vi "YKPZ400 Main.vi"(8 "error in (no error)":errorcluster, 9 "Metadata all":T1={"Data Fields"={"operatorName"="LED Life Testing", "project"="LED Life Testing", "measurementType"="", "sphere"="2m (jacketed)", "spectrometer"="", "powerSource"="California Instruments 2253ix", "analyzer"="California Instruments 2253ix", "fixtureType"="NA", "lampType"="A 19", "sourceType"="LED", "testOrientation"="Base Up", "model"="1", "sample"="1", "hours"="1000", "Amp Gain Range"=""}, "Metadata Disable"={"spectrometer"=enum."Disabled and Grayed Out", "sphere"=enum."Disabled and Grayed Out", "analyzer"=enum."Disabled and Grayed Out", "ampGainRange"=enum."Disabled and Grayed Out"}, "Output Path"=path ""}, 10 "Master":refnum<queue>, 11 "Stand alone?":bool) -> (0 "error out":errorcluster)   [LabVIEW 2013, in "Yokogawa.lvlib"]
doc: "This Continuous Measurement sample project is based on the Queued Message Handler template.\n\nThe Event Handling Loop generates messages based on user interface actions.\n\nThe Message Handling Loop processes messages generated by the Event Handling Loop, or by other messages. There are also Acquisition and Logging message handling loop subVIs, and a chart updating loop."
uses:
  Yokogawa.lvlib
  controls/electrical2.ctl
  support/Message Queue/Message Cluster.ctl
  controls/Metadata all typedef.ctl
  controls/Metadata typedef.ctl
  controls/Metadata disable typedef.ctl
  Settings/Settings.ctl
  Acquisition/Hardware Configuration.ctl
  Logging/Logging Configuration.ctl
  controls/YKPZ400 UI Data.ctl
  controls/YKPZ400 UI State.ctl
  support/Message Queue/Enqueue Message (Single).vi
  support/Message Queue/Enqueue Message (Array).vi
  <vilib>/Utility/error.llb/Error Cluster From Error Code.vi
  <vilib>/ErrorRing/Error Ring.xnode
  Acquisition/YKPZ400 Acquisition.lvlib
  Logging/YKPZ400 Logging.lvlib
  Settings/YKPZ400 Settings.lvlib
  support/User Event - Stop/YKPZ400 User Event - Stop.lvlib
  support/Message Queue/YKPZ400 Message Queue.lvlib
panel:
  out "Electrical Data":T4
  in  "Save Data":bool
  in  "Settings":bool
  in  "Start":bool
  in  "Stop":bool
  in  "Exit":bool
  out "Status":string
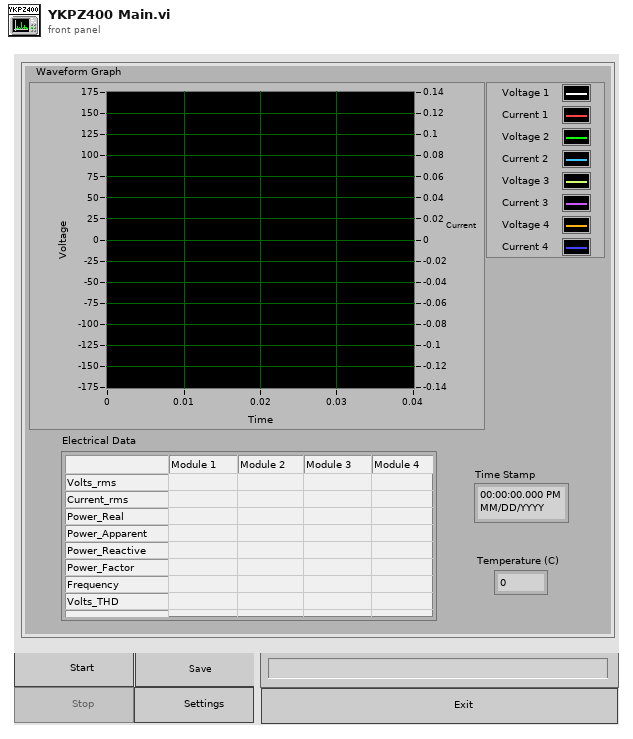
[diagram p1: front panel]
types:
  T1 = typedef "Yokogawa.lvlib/YKPZ400 Logging.lvlib/Metadata all typedef.ctl" = cluster{"Data Fields":T2, "Metadata Disable":T3, "Output Path":path}
  T2 = typedef "Yokogawa.lvlib/YKPZ400 Logging.lvlib/Metadata typedef.ctl" = cluster{"operatorName":string, "project":string, "measurementType":string, "sphere":string, "spectrometer":string, "powerSource":string, "analyzer":string, "fixtureType":string, "lampType":string, "sourceType":string, "testOrientation":string, "model":string, "sample":string, "hours":string, "Amp Gain Range":string}
  T3 = typedef "Yokogawa.lvlib/YKPZ400 Logging.lvlib/Metadata disable typedef.ctl" = cluster{"spectrometer":enum8{"Enabled", "Disabled", "Disabled and Grayed Out"}, "sphere":enum8{"Enabled", "Disabled", "Disabled and Grayed Out"}, "analyzer":enum8{"Enabled", "Disabled", "Disabled and Grayed Out"}, "ampGainRange":enum8{"Enabled", "Disabled", "Disabled and Grayed Out"}}
  T4 = typedef "Yokogawa.lvlib/YKPZ400 Acquisition.lvlib/electrical2.ctl" = cluster{"Time Stamp":timestamp, "Temperature (C)":dbl, "Electrical Data":string[][], "Waveform Graph":waveform(dbl)[]}
  T5 = typedef "Yokogawa.lvlib/YKPZ400 UI State.ctl" = enum16{"Idle", "Acquiring and Logging", "Waiting for Exit", "Waiting for Exit (Acq Stopped)", "Waiting for Exit (Log Stopped)", "Waiting for Stop", "Waiting for Stop (Acq Stopped)", "Waiting for Stop (Log Stopped)"}
  T6 = typedef "Yokogawa.lvlib/YKPZ400 UI Data.ctl" = cluster{"Start Ref":refnum<vi>, "Stop Ref":refnum<vi>, "Settings Ref":refnum<vi>, "Exit Ref":refnum<vi>, "Status Ref":refnum<vi>, "Clust Refnum":refnum<vi>, "Save Refnum":refnum<vi>}
  T7 = typedef "Yokogawa.lvlib/YKPZ400 Settings.lvlib/Settings.ctl" = cluster{"Hardware Configuration":T8, "Logging Configuration":T9}
  T8 = typedef "Yokogawa.lvlib/YKPZ400 Acquisition.lvlib/Hardware Configuration.ctl" = cluster{"VISA resource name":refnum<visa-resource-name>, "Mode (0: Normal) ":u16, "Voltage":cluster{"Element (0: All)":u16, "V Range (200)":u16}, "Current":cluster{"A Range (2)":u16, "A Terminal (0: 5A)":u16, "Element (0: ALL)":u16}, "Observation Time":u16, "Modules on/off":cluster{"Module 1":bool, "Module 2":bool, "Module 3":bool, "Module 4":bool}}
  T9 = typedef "Yokogawa.lvlib/YKPZ400 Logging.lvlib/Logging Configuration.ctl" = cluster{"Log File Base Path":path, "TDMS File Reference":refnum<k34>, "Module to save":i32}
  T10 = typedef "Yokogawa.lvlib/YKPZ400 Message Queue.lvlib/All Message Queues.ctl" = cluster{"Master":refnum<queue>, "UI":refnum<queue>, "Acquisition":refnum<queue>, "Logging":refnum<queue>}
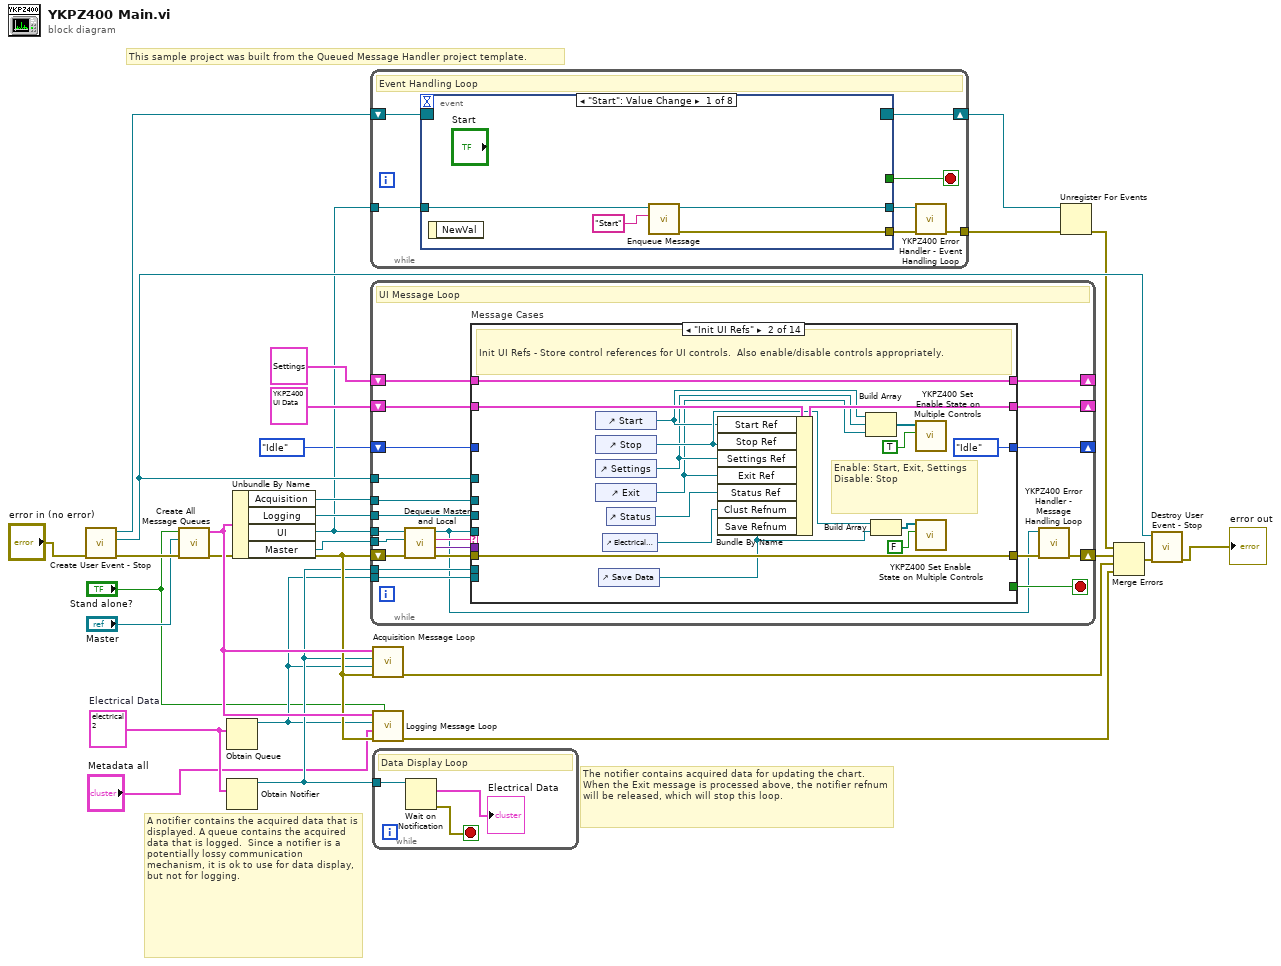
[diagram p0: block diagram]
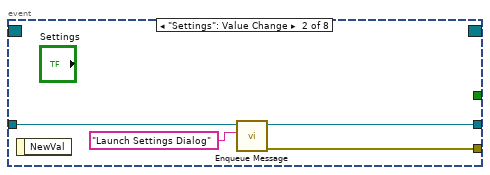
[diagram p2: hidden frame]
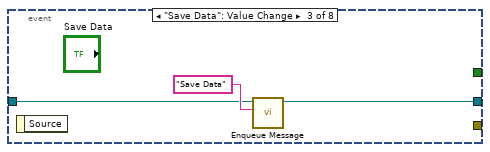
[diagram p3: hidden frame]
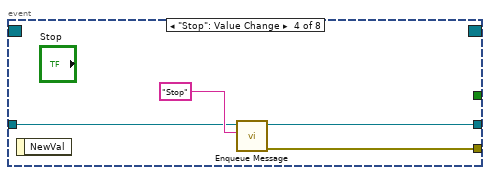
[diagram p4: hidden frame]
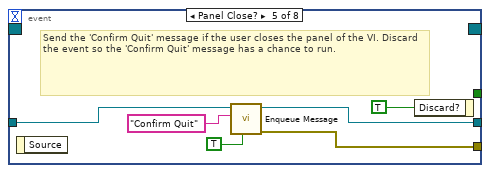
[diagram p5: hidden frame]
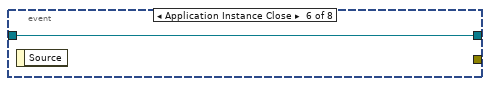
[diagram p6: hidden frame]
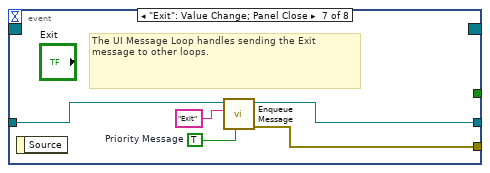
[diagram p7: hidden frame]
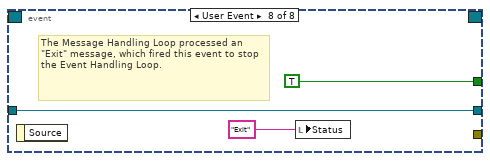
[diagram p8: hidden frame]
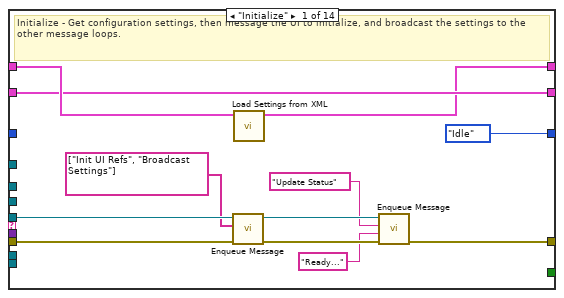
[diagram p9: hidden frame]
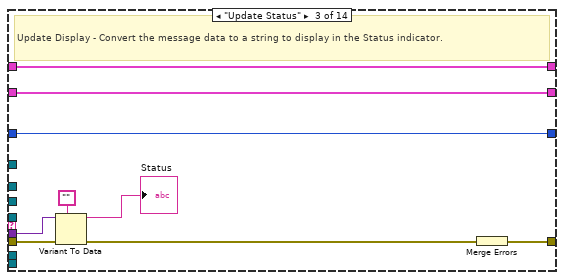
[diagram p10: hidden frame]
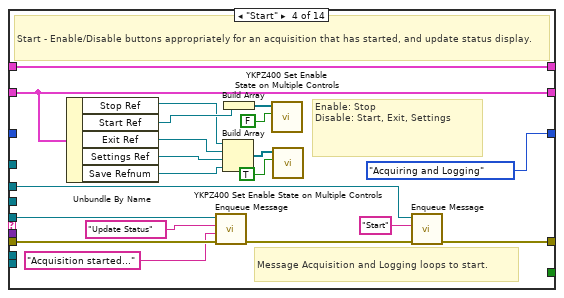
[diagram p11: hidden frame]
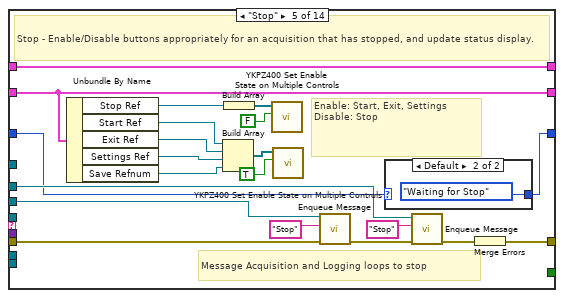
[diagram p12: hidden frame]
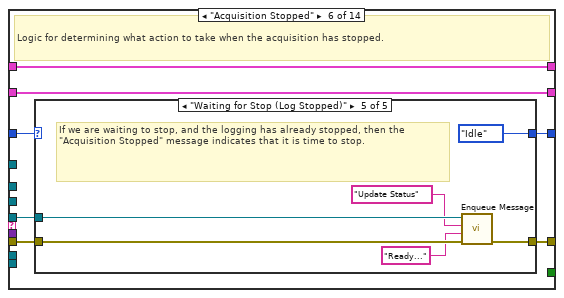
[diagram p14: hidden frame]
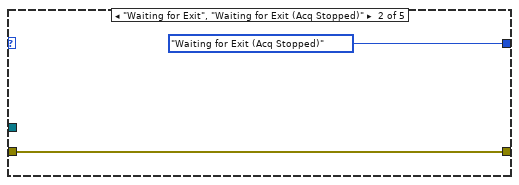
[diagram p16: hidden frame]
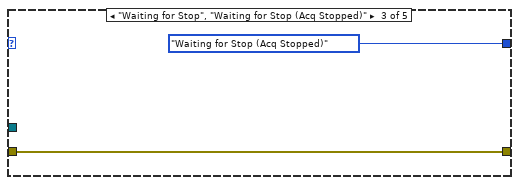
[diagram p17: hidden frame]
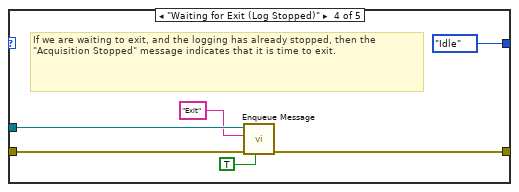
[diagram p18: hidden frame]
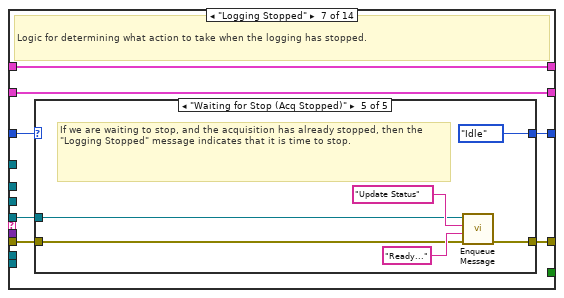
[diagram p19: hidden frame]
diagram:
  w9 = T4 {"Time Stamp"=timestamp(0 s since 1904-01-01), "Temperature (C)"=0.0, "Electrical Data"=[], "Waveform Graph"=[]}  # Electrical Data
  # "This sample project was built from the Queued Message Handler project template."
  # "A notifier contains the acquired data that is displayed. A queue contains the acquired data that is logged.  Since a notifier is a potentially lossy communication mechanism, it is ok to use for data display, but not for logging."
  # "The notifier contains acquired data for updating the chart. When the Exit message is processed above, the notifier refnum will be released, which will stop this loop."
  n1 = call "Create User Event - Stop.vi"("error in (no error)"="error in (no error)") -> ("error out"=w22:errorcluster, "User Event - Stop"=w24:refnum<user-event>, "Stop Event Registration Refnum"=w25:refnum<event-registration>)  [unwired: 8 in]
  n2 = call "Create All Message Queues.vi"("error in (no error)"=w22, "Master"="Master", "Stand alone?"="Stand alone?") -> ("error out"=w19:errorcluster, "Message Queues out"=w21:T10)  [unwired: 7 in]
  n3 = Obtain Queue(element data type=w9) -> (queue out=w7:refnum<queue>)  [unwired: 4 in, 2 out]
  n4 = Obtain Notifier(notification data type=w9) -> (notifier out=w8:refnum<notifier>)  [unwired: 3 in, 2 out]
  n5 = Unbundle By Name(w21) -> ("Acquisition"=w14:refnum<queue>, "Logging"=w13:refnum<queue>, "UI"=w12:refnum<queue>, "Master"=w1:refnum<queue>)
  n6 = while {
    tunnel: w12 -> [w33]
    tunnel: [w30] -> w26
    shift-right: [w32] -> w16
    shift-left: w25 -> [w34]
    stop <- w31 stop-if-true
    # "Event Handling Loop"
    n7 = event shown="[0] \"Start\": Value Change" {
      selector: w34 -> [_ _ _ _ _ _ _ _]
      dyn-events: [_ _ _ _ _ _ _ _] -> w32
      timeout: _ -> [_ _ _ _ _ _ _ _]
      tunnel: [_ _ _ _ _ _ _ TRUE ("Discard?")] -> w31
      tunnel: w33 -> [w38 w40 w44 w48 w53 w56 w58 w62]
      tunnel: [w36 w42 _ w47 w51 _ w61 _] -> w29
      tunnel: [w35 w39 w43 w46 w52 w56 w57 w62] -> w28
      event "Start": Value Change {
        n8 = event-data() -> ()  [unwired: 1 in, 1 out]
        n9 = call-poly "Enqueue Message.vi"("Message"="Start", "Message Queue"=w38) -> ("error out"=w36:errorcluster, "dup Message Queue"=w35:refnum<queue>)  [unwired: 8 in]
      }
      event "Settings": Value Change {
        n10 = event-data() -> ()  [unwired: 1 in, 1 out]
        n11 = call-poly "Enqueue Message.vi"("Message"="Launch Settings Dialog", "Message Queue"=w40) -> ("error out"=w42:errorcluster, "dup Message Queue"=w39:refnum<queue>)  [unwired: 8 in]
      }
      event "Save Data": Value Change {
        n12 = event-data() -> ()  [unwired: 1 in, 1 out]
        n13 = call-poly "Enqueue Message.vi"("Message"="Save Data", "Message Queue"=w44) -> ("dup Message Queue"=w43:refnum<queue>)  [unwired: 8 in, 1 out]
      }
      event "Stop": Value Change {
        n14 = event-data() -> ()  [unwired: 1 in, 1 out]
        n15 = call-poly "Enqueue Message.vi"("Message"="Stop", "Message Queue"=w48) -> ("error out"=w47:errorcluster, "dup Message Queue"=w46:refnum<queue>)  [unwired: 8 in]
      }
      event Panel Close? {
        # "Send the 'Confirm Quit' message if the user closes the panel of the VI. Discard the event so the 'Confirm Quit' message has a chance to run."
        n16 = event-data() -> ()  [unwired: 1 in, 1 out]
        n17 = call-poly "Enqueue Message.vi"("Priority Message? (F)"=TRUE, "Message"="Confirm Quit", "Message Queue"=w53) -> ("error out"=w51:errorcluster, "dup Message Queue"=w52:refnum<queue>)  [unwired: 7 in]
        n18 = event-data("Discard?"=TRUE) -> ()  [unwired: 1 in, 1 out]
      }
      event Application Instance Close {
        n19 = event-data() -> ()  [unwired: 1 in, 1 out]
      }
      event "Exit": Value Change; Panel Close {
        w59 = TRUE  # Priority Message
        # "The UI Message Loop handles sending the Exit message to other loops."
        n20 = event-data() -> ()  [unwired: 1 in, 1 out]
        n21 = call-poly "Enqueue Message.vi"("Priority Message? (F)"=w59, "Message"="Exit", "Message Queue"=w58) -> ("error out"=w61:errorcluster, "dup Message Queue"=w57:refnum<queue>)  [unwired: 7 in]
      }
      event User Event {
        # "The Message Handling Loop processed an \"Exit\" message, which fired this event to stop the Event Handling Loop."
        n22 = event-data() -> ()  [unwired: 1 in, 1 out]
        n23 = local write "Status"("Exit" ("Exit String")) -> ()
      }
    }
    n24 = call "YKPZ400 Error Handler - Event Handling Loop.vi"("error in (no error)"=w29, "Message Queue"=w28) -> ("dup error in"=w30:errorcluster)  [unwired: 8 in, 1 out]
  }
  n25 = while {
    tunnel: w12 -> [w71]
    tunnel: w24 -> [w84]
    shift-right: [w75] -> w27
    shift-left: w19 -> [w69]
    shift-right: [w83] -> _
    shift-left: T7 {"Hardware Configuration"={"VISA resource name"="", "Mode (0: Normal) "=0, "Voltage"={"Element (0: All)"=0, "V Range (200)"=0}, "Current"={"A Range (2)"=0, "A Terminal (0: 5A)"=0, "Element (0: ALL)"=0}, "Observation Time"=0, "Modules on/off"={"Module 1"=FALSE, "Module 2"=FALSE, "Module 3"=FALSE, "Module 4"=FALSE}}, "Logging Configuration"={"Log File Base Path"=path "", "TDMS File Reference"=refnum, "Module to save"=0}} ("Settings") -> [w82]
    shift-right: [w80] -> _
    shift-left: T6 {"Start Ref"=refnum, "Stop Ref"=refnum, "Settings Ref"=refnum, "Exit Ref"=refnum, "Status Ref"=refnum, "Clust Refnum"=refnum, "Save Refnum"=refnum} ("Measurement UI Controls") -> [w81]
    tunnel: w14 -> [w79]
    tunnel: w13 -> [w78]
    tunnel: w8 -> [w77]
    tunnel: w7 -> [w76]
    shift-right: [w72] -> _
    shift-left: YKPZ400_UI_State."Idle" ("UI State") -> [w73]
    tunnel: w1 -> [w70]
    stop <- w85 stop-if-true
    # "UI Message Loop"
    n26 = call "Dequeue Master and Local.vi"("error in (no error)"=w69, "Master"=w70, "UI In"=w71) -> ("error out"=w67:errorcluster, "Message Data"=w68:variant, "Message"=w66:string, "UI Out"=w65:refnum<queue>)  [unwired: 5 in]
    n27 = case "Message Cases" shown="\"Init UI Refs\"" w66 {
      selector: w66 -> [_ _ _ _ _ _ _ _ _ _ _ _ _ w313]
      tunnel: w65 -> [w90 _ _ w142 _ w168 w193 _ w233 w247 w258 w289 w303 _]
      tunnel: w67 -> [w89 w113 w121 w141 w162 w169 w194 w221 w235 w250 w257 w297 w301 _]
      tunnel: [w94 w113 w122 w130 w163 w166 w191 w227 w230 w246 w256 w298 w311 w312] -> w74
      tunnel: [_ _ _ _ _ _ _ _ _ _ _ TRUE _ _] -> w85
      tunnel: w68 -> [_ _ w120 _ _ _ _ _ _ w248 _ _ _ _]
      tunnel: w84 -> [_ _ _ _ _ _ _ _ _ _ _ w296 _ _]
      tunnel: [w86 w112 w116 w140 w161 w172 w197 w225 w232 w254 w261 w294 w310 w316] -> w83
      tunnel: w82 -> [w97 w112 w116 w140 w161 w172 w197 w225 w236 w254 w261 w294 w310 w316]
      tunnel: w81 -> [w91 w111 w115 w137 w160 w171 w196 w219 w229 w253 w260 w292 w309 w315]
      tunnel: [w91 w109 w115 w137 w160 w171 w196 w219 w229 w253 w260 w292 w309 w315] -> w80
      tunnel: w79 -> [_ _ _ w129 w147 _ _ w218 _ _ _ w291 _ _]
      tunnel: w78 -> [_ _ _ _ w150 _ _ w217 _ _ _ w290 w306 _]
      tunnel: w77 -> [_ _ _ _ _ _ _ _ _ _ _ w288 _ _]
      tunnel: w76 -> [_ _ _ _ _ _ _ _ _ _ _ w284 _ _]
      tunnel: w73 -> [_ _ w114 _ w144 w170 w195 w216 w228 w242 w259 _ w308 w314]
      tunnel: [YKPZ400_UI_State."Idle" ("UI State") YKPZ400_UI_State."Idle" ("UI State") w114 YKPZ400_UI_State."Acquiring and Logging" ("UI State") w145 w167 w192 w216 w228 w242 w255 YKPZ400_UI_State."Idle" ("UI State") w308 w314] -> w72
      frame "Initialize" {
        # "Initialize - Get configuration settings, then message the UI to initialize, and broadcast the settings to the other message loops."
        n28 = call-poly "Enqueue Message.vi"("error in (no error)"=w89, "Message Array"=string[] ["Init UI Refs", "Broadcast Settings"], "Message Queue"=w90) -> ("error out"=w96:errorcluster, "dup Message Queue"=w95:refnum<queue>)  [unwired: 7 in]
        n29 = call "Load Settings from XML.vi"("Settings in"=w97) -> ("Settings out"=w86:T7)  [unwired: 9 in, 1 out]
        n30 = call-poly "Enqueue Message.vi"("error in (no error)"=w96, "Message Data"="Ready..." ("Ready..."), "Message"="Update Status", "Message Queue"=w95) -> ("error out"=w94:errorcluster)  [unwired: 6 in, 1 out]
      }
      frame "Init UI Refs" {
        # "Enable: Start, Exit, Settings\nDisable: Stop"
        # "Init UI Refs - Store control references for UI controls.  Also enable/disable controls appropriately."
        n31 = control-ref of="Start"() -> (w103:refnum<vi>)
        n32 = control-ref of="Stop"() -> (w104:refnum<vi>)
        n33 = control-ref of="Settings"() -> (w102:refnum<vi>)
        n34 = control-ref of="Exit"() -> (w101:refnum<vi>)
        n35 = control-ref of="Save Data"() -> (w98:refnum<vi>)
        n36 = control-ref of="Electrical Data 2"() -> (w99:refnum<vi>)
        n37 = control-ref of="Status"() -> (w110:refnum<vi>)
        n38 = Bundle By Name(cluster=w111, "Start Ref"=w103, "Stop Ref"=w104, "Settings Ref"=w102, "Exit Ref"=w101, "Status Ref"=w110, "Clust Refnum"=w99, "Save Refnum"=w98) -> (w109:T6)
        n39 = Build Array(w103, w102, w101) -> (w107:refnum<vi>[])
        n40 = Build Array(w104, w98) -> (w106:refnum<vi>[])
        n41 = call "YKPZ400 Set Enable State on Multiple Controls.vi"("Enable?"=TRUE, "Controls"=w107) -> ()  [unwired: 10 in]
        n42 = call "YKPZ400 Set Enable State on Multiple Controls.vi"("Enable?"=FALSE, "Controls"=w106) -> ()  [unwired: 10 in]
      }
      frame "Update Status" {
        # "Update Display - Convert the message data to a string to display in the Status indicator."
        n43 = Variant To Data(error in=w121, type="", Variant=w120) -> (data=→"Status":string, error out=w118:errorcluster)
        n44 = Merge Errors(w118) -> (w122:errorcluster)
      }
      frame "Start" {
        # "Message Acquisition and Logging loops to start."
        # "Enable: Stop\nDisable: Start, Exit, Settings"
        # "Start - Enable/Disable buttons appropriately for an acquisition that has started, and update status display."
        n45 = Unbundle By Name(w137) -> ("Stop Ref"=w123:refnum<vi>, "Start Ref"=w124:refnum<vi>, "Exit Ref"=w132:refnum<vi>, "Settings Ref"=w131:refnum<vi>, "Save Refnum"=w125:refnum<vi>)
        n46 = call-poly "Enqueue Message.vi"("error in (no error)"=w141, "Message Data"="Acquisition started..." ("Acquiring and Logging..."), "Message"="Update Status", "Message Queue"=w142) -> ("error out"=w126:errorcluster)  [unwired: 6 in, 1 out]
        n47 = Build Array(w123, w132, w131, w125) -> (w135:refnum<vi>[])
        n48 = Build Array(w124) -> (w134:refnum<vi>[])
        n49 = call "YKPZ400 Set Enable State on Multiple Controls.vi"("Enable?"=FALSE, "Controls"=w134) -> ()  [unwired: 10 in]
        n50 = call "YKPZ400 Set Enable State on Multiple Controls.vi"("Enable?"=TRUE, "Controls"=w135) -> ()  [unwired: 10 in]
        n51 = call-poly "Enqueue Message.vi"("error in (no error)"=w126, "Message"="Start", "Message Queue"=w129) -> ("error out"=w130:errorcluster)  [unwired: 7 in, 1 out]
      }
      frame "Stop" {
        # "Message Acquisition and Logging loops to stop"
        # "Enable: Start, Exit, Settings\nDisable: Stop"
        # "Stop - Enable/Disable buttons appropriately for an acquisition that has stopped, and update status display."
        n52 = Unbundle By Name(w160) -> ("Stop Ref"=w155:refnum<vi>, "Start Ref"=w154:refnum<vi>, "Exit Ref"=w153:refnum<vi>, "Settings Ref"=w152:refnum<vi>, "Save Refnum"=w143:refnum<vi>)
        n53 = Build Array(w154, w153, w152, w143) -> (w158:refnum<vi>[])
        n54 = Build Array(w155) -> (w157:refnum<vi>[])
        n55 = call "YKPZ400 Set Enable State on Multiple Controls.vi"("Enable?"=FALSE, "Controls"=w157) -> ()  [unwired: 10 in]
        n56 = call "YKPZ400 Set Enable State on Multiple Controls.vi"("Enable?"=TRUE, "Controls"=w158) -> ()  [unwired: 10 in]
        n57 = call-poly "Enqueue Message.vi"("error in (no error)"=w162, "Message"="Stop", "Message Queue"=w150) -> ("error out"=w149:errorcluster)  [unwired: 7 in, 1 out]
        n58 = case shown="Default" w144 {
          selector: w144 -> [w164 _]
          tunnel: [w164 YKPZ400_UI_State."Waiting for Stop" ("UI State")] -> w145
          frame "Waiting for Exit" {
          }
          frame Default {
          }
        }
        n59 = call-poly "Enqueue Message.vi"("error in (no error)"=w149, "Message"="Stop", "Message Queue"=w147) -> ("error out"=w148:errorcluster)  [unwired: 7 in, 1 out]
        n60 = Merge Errors(w148) -> (w163:errorcluster)
      }
      frame "Acquisition Stopped" {
        # "Logic for determining what action to take when the acquisition has stopped."
        n61 = case shown="\"Waiting for Stop (Log Stopped)\"" w170 {
          selector: w170 -> [w174 _ _ _ _]
          tunnel: w169 -> [w173 w176 w178 w184 w190]
          tunnel: w168 -> [_ _ _ w182 w187]
          tunnel: [w174 YKPZ400_UI_State."Waiting for Exit (Acq Stopped)" ("UI State") YKPZ400_UI_State."Waiting for Stop (Acq Stopped)" ("UI State") YKPZ400_UI_State."Idle" ("UI State") YKPZ400_UI_State."Idle" ("UI State")] -> w167
          tunnel: [w173 w176 w178 w183 w188] -> w166
          frame Default {
          }
          frame "Waiting for Exit", "Waiting for Exit (Acq Stopped)" {
          }
          frame "Waiting for Stop", "Waiting for Stop (Acq Stopped)" {
          }
          frame "Waiting for Exit (Log Stopped)" {
            # "If we are waiting to exit, and the logging has already stopped, then the \"Acquisition Stopped\" message indicates that it is time to exit."
            n62 = call-poly "Enqueue Message.vi"("Priority Message? (F)"=TRUE, "error in (no error)"=w184, "Message"="Exit", "Message Queue"=w182) -> ("error out"=w183:errorcluster)  [unwired: 6 in, 1 out]
          }
          frame "Waiting for Stop (Log Stopped)" {
            # "If we are waiting to stop, and the logging has already stopped, then the \"Acquisition Stopped\" message indicates that it is time to stop."
            n63 = call-poly "Enqueue Message.vi"("error in (no error)"=w190, "Message Data"="Ready..." ("Ready..."), "Message"="Update Status", "Message Queue"=w187) -> ("error out"=w188:errorcluster)  [unwired: 6 in, 1 out]
          }
        }
      }
      frame "Logging Stopped" {
        # "Logic for determining what action to take when the logging has stopped."
        n64 = case shown="\"Waiting for Stop (Acq Stopped)\"" w195 {
          selector: w195 -> [w199 _ _ _ _]
          tunnel: w194 -> [w198 w201 w203 w209 w212]
          tunnel: w193 -> [_ _ _ w207 w211]
          tunnel: [w199 YKPZ400_UI_State."Waiting for Exit (Log Stopped)" ("UI State") YKPZ400_UI_State."Waiting for Stop (Log Stopped)" ("UI State") YKPZ400_UI_State."Idle" ("UI State") YKPZ400_UI_State."Idle" ("UI State")] -> w192
          tunnel: [w198 w201 w203 w208 w210] -> w191
          frame Default {
          }
          frame "Waiting for Exit", "Waiting for Exit (Log Stopped)" {
          }
          frame "Waiting for Stop", "Waiting for Stop (Log Stopped)" {
          }
          frame "Waiting for Exit (Acq Stopped)" {
            # "If we are waiting to exit, and the acquisition has already stopped, then the \"Logging Stopped\" message indicates that it is time to exit."
            n65 = call-poly "Enqueue Message.vi"("Priority Message? (F)"=TRUE, "error in (no error)"=w209, "Message"="Exit", "Message Queue"=w207) -> ("error out"=w208:errorcluster)  [unwired: 6 in, 1 out]
          }
          frame "Waiting for Stop (Acq Stopped)" {
            # "If we are waiting to stop, and the acquisition has already stopped, then the \"Logging Stopped\" message indicates that it is time to stop."
            n66 = call-poly "Enqueue Message.vi"("error in (no error)"=w212, "Message Data"="Ready..." ("Ready..."), "Message"="Update Status", "Message Queue"=w211) -> ("error out"=w210:errorcluster)  [unwired: 6 in, 1 out]
          }
        }
      }
      frame "Broadcast settings" {
        w220 = "Update Settings" ("Message")
        # "Broadcast settings - Send the 'Update Settings' message to the Logging and Acquisition message loops."
        n67 = Unbundle By Name(w225) -> ("Hardware Configuration"=w224:T8, "Logging Configuration"=w223:T9)
        n68 = call-poly "Enqueue Message.vi"("Message Data"=w224, "Message"=w220, "Message Queue"=w218) -> ("error out"=w226:errorcluster)  [unwired: 7 in, 1 out]
        n69 = call-poly "Enqueue Message.vi"("error in (no error)"=w226, "Message Data"=w223, "Message"=w220, "Message Queue"=w217) -> ("error out"=w222:errorcluster)  [unwired: 6 in, 1 out]
        n70 = Merge Errors(w222, w221) -> (w227:errorcluster)
      }
      frame "Launch Settings Dialog" {
        # "Launch Settings Dialog - Launch the Settings Dialog when the user clicks the 'Settings' button."
        n71 = call "Settings Dialog.vi"("error in (no error)"=w235, "Settings in"=w236) -> ("error out"=w231:errorcluster, "Cancelled?"=w234:bool, "Settings out"=w232:T7)  [unwired: 6 in, 1 out]
        n72 = case shown="False" w234 {
          tunnel: w233 -> [w240 _]
          tunnel: w231 -> [w239 w241]
          tunnel: [w238 w241] -> w230
          frame False {
            n73 = call-poly "Enqueue Message.vi"("error in (no error)"=w239, "Message"="Broadcast Settings", "Message Queue"=w240) -> ("error out"=w238:errorcluster)  [unwired: 7 in, 1 out]
          }
          frame True {
          }
        }
      }
      frame "Error" {
        # "Error - Check the error message data and respond accordingly. This message is sent by the \"Error Handler\" VIs at the end of each loop in this application."
        n74 = Variant To Data(error in=w250, type=errorcluster {"status"=FALSE, "code"=0, "source"=""} ("error constant"), Variant=w248) -> (data=w252:errorcluster, error out=w249:errorcluster)
        n75 = call <vilib>:"Simple Error Handler.vi"("error in (no error)"=w252) -> ()  [unwired: 4 in, 5 out]
        n76 = call-poly "Enqueue Message.vi"("Priority Message? (F)"=TRUE, "Message"="Exit", "Message Queue"=w247) -> ("error out"=w245:errorcluster)  [unwired: 7 in, 1 out]
        n77 = Merge Errors(w245, w249) -> (w246:errorcluster)
      }
      frame "Confirm Quit" {
        # "Confirm Quit - Message that can confirm whether or not the user wants to exit the application."
        n78 = case shown="\"Acquiring and Logging\"" w259 {
          tunnel: w258 -> [w267 w271]
          tunnel: w257 -> [w266 w270]
          tunnel: [w265 w269] -> w256
          tunnel: [YKPZ400_UI_State."Idle" ("UI State") w268] -> w255
          frame Default {
            # "If 'Confirm Quit' comes in while the system is idle, there is no need for a confirmation message."
            n79 = call-poly "Enqueue Message.vi"("Priority Message? (F)"=TRUE, "error in (no error)"=w266, "Message"="Exit", "Message Queue"=w267) -> ("error out"=w265:errorcluster)  [unwired: 6 in, 1 out]
          }
          frame "Acquiring and Logging" {
            n80 = Two Button Dialog(message="Are you sure you want to quit while the acquisition is running?" ("Confirm Quit Message"), 1:"No" ("No"), 2:"Yes" ("Yes")) -> (T button?=w272:bool)
            n81 = case shown="True" w272 {
              tunnel: w271 -> [_ w281]
              tunnel: w270 -> [w277 w282]
              tunnel: [w277 w280] -> w269
              tunnel: [YKPZ400_UI_State."Acquiring and Logging" ("UI State") YKPZ400_UI_State."Waiting for Exit" ("UI State")] -> w268
              frame False {
                # "User did not want to quit."
              }
              frame True {
                n82 = call-poly "Enqueue Message.vi"("error in (no error)"=w282, "Message"="Stop", "Message Queue"=w281) -> ("error out"=w280:errorcluster)  [unwired: 7 in, 1 out]
              }
            }
          }
        }
      }
      frame "Exit" {
        w293 = "Exit" ("Message")
        # "Don't check the error outs. The acquisition and logging queues may have already been released."
        # "Close references owned by the Main VI."
        # "Stop the VI"
        # "Exit - Fire the User Event to stop the Event Handling Loop.  Also send Exit messages to the Acquisition and Logging loops."
        n83 = Release Queue(queue=w289, error in (no error)=w297) -> (error out=w287:errorcluster)  [unwired: 1 in, 2 out]
        n84 = call "Fire User Event - Stop.vi"("User Event - Stop"=w296) -> ("error out"=w295:errorcluster)  [unwired: 10 in]
        n85 = Release Notifier(notifier=w288, error in (no error)=w287) -> (error out=w286:errorcluster)  [unwired: 1 in, 2 out]
        n86 = Release Queue(queue=w284, error in (no error)=w286) -> (error out=w285:errorcluster)  [unwired: 1 in, 2 out]
        n87 = call-poly "Enqueue Message.vi"("Message"=w293, "Message Queue"=w291) -> ()  [unwired: 8 in, 2 out]
        n88 = call-poly "Enqueue Message.vi"("Message"=w293, "Message Queue"=w290) -> ()  [unwired: 8 in, 2 out]
        n89 = Merge Errors(w295, w285) -> (w298:errorcluster)
      }
      frame "Save Data" {
        # "Duplicate this frame when creating new messages.  Change this comment in the duplicated frame to describe this message."
        n90 = call-poly "Enqueue Message.vi"("error in (no error)"=w301, "Message Data"="Saving Data..." ("Message"), "Message"="Update Status", "Message Queue"=w303) -> ("error out"=w300:errorcluster)  [unwired: 6 in, 1 out]
        n91 = call-poly "Enqueue Message.vi"("error in (no error)"=w300, "Message"="Single Log", "Message Queue"=w306) -> ("error out"=w305:errorcluster)  [unwired: 7 in, 1 out]
        n92 = Merge Errors(w305) -> (w311:errorcluster)
      }
      frame Default {
        # "'Default' case only runs if there is a message that isn't defined in any of the other cases.  Output a programming error."
        n93 = xnode "Error Ring"("parameter 0"=w313) -> ("error out"=w312:errorcluster)
      }
    }
    n94 = call "YKPZ400 Error Handler - Message Handling Loop.vi"("error in (no error)"=w74, "Message Queue"=w65) -> ("dup error in"=w75:errorcluster)  [unwired: 8 in, 1 out]
  }
  n95 = call "Acquisition Message Loop.vi"("error in (no error)"=w19, "Data Queue 2"=w7, "Data Notifier 2"=w8, "Message Queues"=w21) -> ("error out"=w23:errorcluster)  [unwired: 7 in]
  n96 = call "Logging Message Loop.vi"("Stand alone?"="Stand alone?", "error in (no error)"=w19, "Metadata all"="Metadata all", "Data Queue"=w7, "Message Queues"=w21) -> ("error out"=w20:errorcluster)  [unwired: 6 in]
  n97 = while "Data Display Loop" {
    tunnel: w8 -> [w326]
    stop <- w325 stop-if-true
    # "Data Display Loop"
    n98 = Wait on Notification(notifier=w326) -> (notification=→"Electrical Data":T4, error out=w325:errorcluster)  [unwired: 3 in, 2 out]
  }
  n99 = Unregister For Events(event registration refnum=w16, error in=w26) -> (error out=w17:errorcluster)
  n100 = Merge Errors(w17, w27, w23, w20) -> (w10:errorcluster)
  n101 = call "Destroy User Event - Stop.vi"("error in (no error)"=w10, "User Event - Stop"=w24) -> ("error out"=→"error out":errorcluster)  [unwired: 9 in]
